vi "CAENHV Get Crate Map.vi"(8 "error in (no error)":errorcluster, 11 "handle":i32) -> (0 "error out":errorcluster, 1 "SerNumList":i16[](array[numeric]), 2 "NrofChList":i16[](array[numeric]), 3 "NrOfSlot":u16, 4 "FmwRelMinList":string[](array[string]), 5 "DescriptionList":string[](array[string]), 6 "FmwRelMaxList":string[](array[string]), 7 "ModelList":string[](array[string]))   [LabVIEW 2009, in "CAENHVWrapper.lvlib"]
doc: "CAENHVLIB_API CAENHVRESULT CAENHV_GetCrateMap(int handle, \n ushort *NrOfSlot, ushort **NrofChList, char **ModelList, char **DescriptionList,\n ushort **SerNumList, uchar **FmwRelMinList, uchar **FmwRelMaxList);"
uses:
  <userlib>/CAENHVWrapper/CAENHVWrapper.lvlib
  <vilib>/Utility/importsl/GetValueByPointer/GetValueByPointer.xnode
  <vilib>/Utility/importsl/GetValueByPointer/datatype.ctl
  <userlib>/CAENHVWrapper/CAENHVWrapper.dll
  resource/lvimptsl.dll
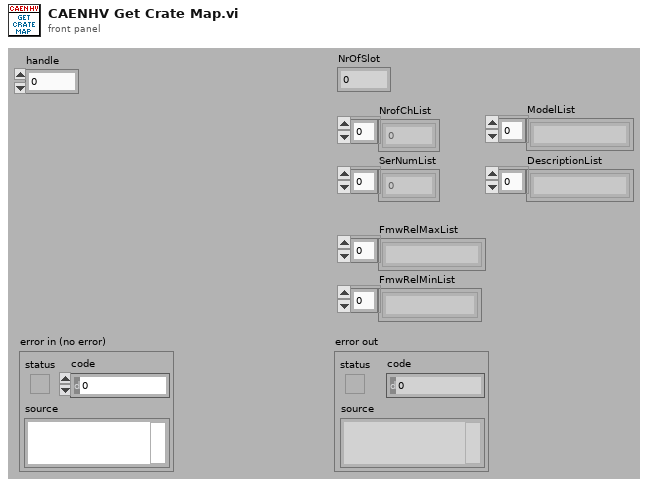
[diagram p1: front panel]
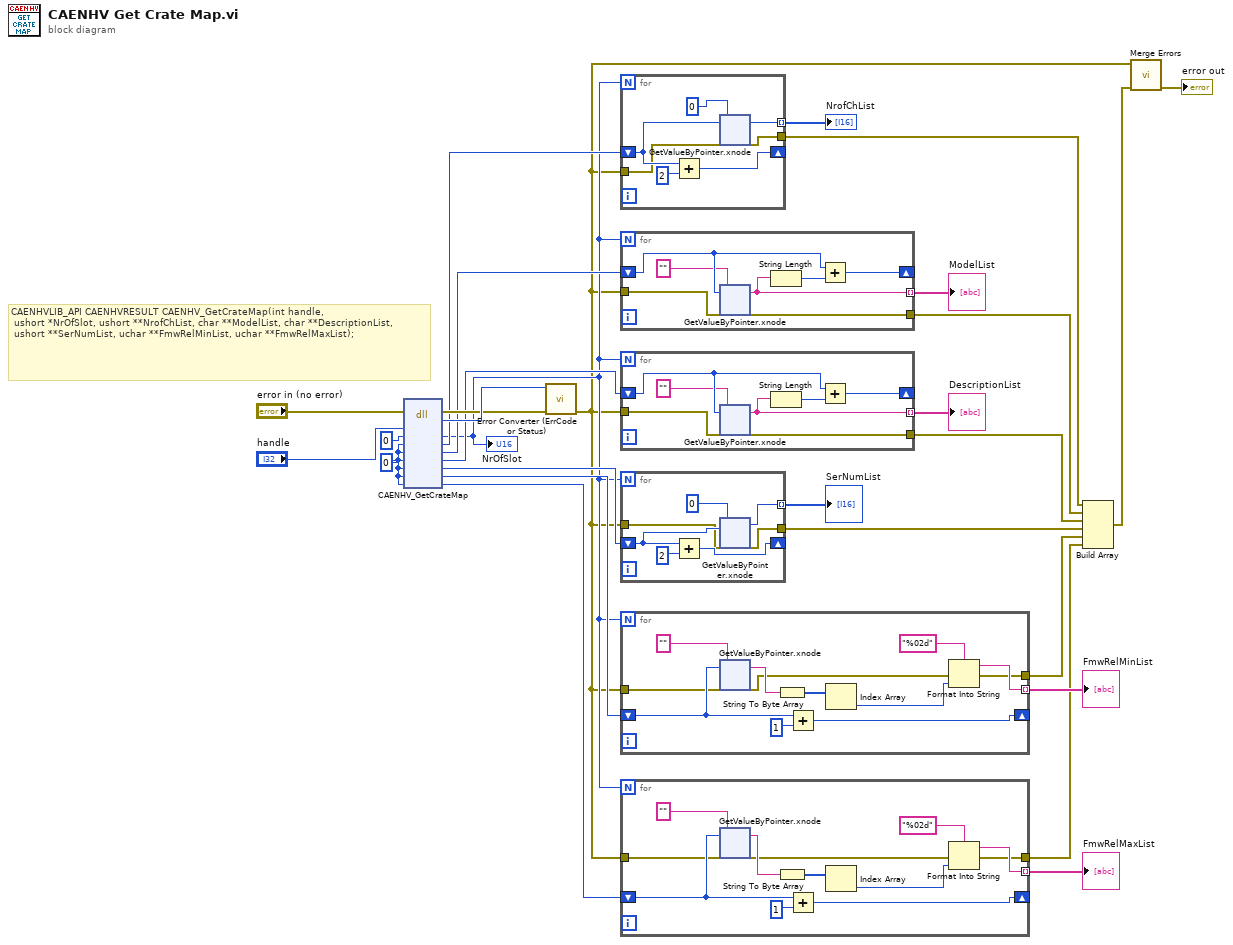
[diagram p0: block diagram]
diagram:
  w23 = i64 0 ("ModelList")
  # "CAENHVLIB_API CAENHVRESULT CAENHV_GetCrateMap(int handle,\t\n ushort *NrOfSlot, ushort **NrofChList, char **ModelList, char **DescriptionList,\n ushort **SerNumList, uchar **FmwRelMinList, uchar **FmwRelMaxList);"
  n1 = dll-call lib="C:/Program Files/National Instruments/LabVIEW 2009/user.lib/CAENHVWrapper/CAENHVWrapper.*" fn="CAENHV_GetCrateMap"(error in="error in (no error)", "handle"="handle", "NrOfSlot"=u16 0, "NrofChList"=w23, "ModelList"=w23, "DescriptionList"=w23, "SerNumList"=w23, "FmwRelMinList"=w23, "FmwRelMaxList"=w23) -> (error out=w24:errorcluster, "return type"=w25:i32, "NrOfSlot"=w12:u16, "NrofChList"=w22:i64, "ModelList"=w21:i64, "DescriptionList"=w16:i64, "SerNumList"=w20:i64, "FmwRelMinList"=w14:i64, "FmwRelMaxList"=w11:i64)  [unwired: 3 in, 1 out]
  "NrOfSlot" <- w12
  n2 = call <userlib>:"Error Converter (ErrCode or Status).vi"("error in (no error)"=w24, "error code"=w25) -> ("error out"=w2:errorcluster)  [unwired: 9 in]
  n3 = for {
    N: w12 -> [_]
    tunnel: [w35] -> w9
    shift-right: [w34] -> _
    shift-left: w22 -> [w31]
    tunnel: [w33] -> w19 mode=indexing
    tunnel: w2 -> [w30]
    n4 = Add(x=w31, y=i64 2) -> (x+y=w34:i64)
    n5 = xnode "GetValueByPointer.xnode"("Pointer"=w31, "InputType"=i16 0, "ErrorIn"=w30) -> ("Output"=w33:i16, "ErrorOut"=w35:errorcluster)  [unwired: 1 in]
  }
  "NrofChList" <- w19
  n6 = for {
    N: w12 -> [_]
    tunnel: [w50] -> w8
    shift-right: [w49] -> _
    shift-left: w21 -> [w48]
    tunnel: [w45] -> w18 mode=indexing
    tunnel: w2 -> [w47]
    n7 = xnode "GetValueByPointer.xnode"("Pointer"=w48, "InputType"="", "ErrorIn"=w47) -> ("Output"=w45:string, "ErrorOut"=w50:errorcluster)  [unwired: 1 in]
    n8 = String Length(string=w45) -> (length=w44:i32)
    n9 = Add(x=w48, y=w44) -> (x+y=w49:i64)
  }
  "ModelList" <- w18
  n10 = for {
    N: w12 -> [_]
    tunnel: [w65] -> w7
    shift-right: [w64] -> _
    shift-left: w16 -> [w63]
    tunnel: [w60] -> w15 mode=indexing
    tunnel: w2 -> [w62]
    n11 = xnode "GetValueByPointer.xnode"("Pointer"=w63, "InputType"="", "ErrorIn"=w62) -> ("Output"=w60:string, "ErrorOut"=w65:errorcluster)  [unwired: 1 in]
    n12 = String Length(string=w60) -> (length=w59:i32)
    n13 = Add(x=w63, y=w59) -> (x+y=w64:i64)
  }
  "DescriptionList" <- w15
  n14 = for {
    N: w12 -> [_]
    tunnel: [w80] -> w6
    shift-right: [w79] -> _
    shift-left: w20 -> [w75]
    tunnel: [w77] -> w17 mode=indexing
    tunnel: w2 -> [w74]
    n15 = Add(x=w75, y=i64 2) -> (x+y=w79:i64)
    n16 = xnode "GetValueByPointer.xnode"("Pointer"=w75, "InputType"=i16 0, "ErrorIn"=w74) -> ("Output"=w77:i16, "ErrorOut"=w80:errorcluster)  [unwired: 1 in]
  }
  "SerNumList" <- w17
  n17 = for {
    N: w12 -> [_]
    shift-right: [w100] -> _
    shift-left: w14 -> [w99]
    tunnel: w2 -> [w98]
    tunnel: [w91] -> w13 mode=indexing
    tunnel: [w89] -> w5
    n18 = xnode "GetValueByPointer.xnode"("Pointer"=w99, "InputType"="", "ErrorIn"=w98) -> ("Output"=w95:string, "ErrorOut"=w90:errorcluster)  [unwired: 1 in]
    n19 = String To Byte Array(string=w95) -> (unsigned byte array=w94:u8[])
    n20 = Add(x=w99, y=i64 1) -> (x+y=w100:i64)
    n21 = Index Array(array=w94) -> (element=w92:u8)  [unwired: 1 in]
    n22 = Format Into String(format string="%02d", error in=w90, w92) -> (resulting string=w91:string, error out=w89:errorcluster)  [unwired: 1 in]
  }
  "FmwRelMinList" <- w13
  n23 = for {
    N: w12 -> [_]
    shift-right: [w120] -> _
    shift-left: w11 -> [w119]
    tunnel: w2 -> [w118]
    tunnel: [w111] -> w10 mode=indexing
    tunnel: [w109] -> w4
    n24 = xnode "GetValueByPointer.xnode"("Pointer"=w119, "InputType"="", "ErrorIn"=w118) -> ("Output"=w115:string, "ErrorOut"=w110:errorcluster)  [unwired: 1 in]
    n25 = String To Byte Array(string=w115) -> (unsigned byte array=w114:u8[])
    n26 = Add(x=w119, y=i64 1) -> (x+y=w120:i64)
    n27 = Index Array(array=w114) -> (element=w112:u8)  [unwired: 1 in]
    n28 = Format Into String(format string="%02d", error in=w110, w112) -> (resulting string=w111:string, error out=w109:errorcluster)  [unwired: 1 in]
  }
  "FmwRelMaxList" <- w10
  n29 = Build Array(w9, w8, w7, w6, w5, w4) -> (w3:errorcluster[])
  n30 = call <vilib>:"Merge Errors.vi"("error array in"=w3, "error in 1 (no error)"=w2) -> ("error out"=→"error out":errorcluster)  [unwired: 5 in]
